vi "Main.vi"(11 "Module Admin":refnum<class "Delacor_lib_QMH_Module Admin.lvclass">) -> ()   [LabVIEW 2018, in "MB 01 switches Module.lvlib"]
doc: "This template is based off of the Queued Message Handler design pattern and the Queued Message Handler project template that ships with LabVIEW.\n\nThe main difference is that the queue is private to this module and communication between modules is performed via Broadcast and Request events.\n\nRequest events are wrapped in public API methods and are handled in the Event Handling Loop (EHL) of this VI. Any module can register for Broadcast events sent by this module. The EHL generates messages based on user interface actions.\n\nThe Message Handling Loop (MHL) processes messages generated by the EHL, or by other messages. The messages are string values, so new messages can be added easily to the Message Cases case structure in the MHL. Each message cluster can also provide an optional value for Message Data, which is a variant that can be converted to whatever message-specific data is required.\n_____\nBased on DQMH Project Template 6.0.0.91."
uses:
  MB 01 switches Module.lvlib
  <vilib>/Delacor/Delacor QMH/Libraries/Module Admin_class/Delacor_lib_QMH_Module Admin.lvclass
  Module Data--cluster.ctl
  <vilib>/NI/Modbus Library/API/Master/Modbus Master.lvclass
  <vilib>/Delacor/Delacor QMH/Libraries/Message Queue_class/Delacor_lib_QMH_Message Queue.lvclass/Delacor_lib_QMH_Message Queue.ctl
  Stop Argument--cluster.ctl
  <vilib>/Delacor/Delacor QMH/Libraries/Module Admin_class/Delacor_lib_QMH_Module Admin.lvclass/Delacor_lib_QMH_Module Admin.ctl
  MB01 Open Argument--cluster.ctl
  demux1-10 Argument--cluster.ctl
  MB01_eMICs Argument--cluster.ctl
  SC enable Argument--cluster.ctl
  MB01 Close Argument--cluster.ctl
  <vilib>/Utility/miscctls.llb/LVPointTypeDef.ctl
  <vilib>/Delacor/Delacor QMH/Libraries/Message Queue_class/Delacor_lib_QMH_Enqueue Message (Single).vi
  <vilib>/Delacor/Delacor QMH/Libraries/Module Admin_class/Delacor_lib_QMH_Get External Launch.vi
  <vilib>/Utility/error.llb/Error Cluster From Error Code.vi
  <vilib>/ErrorRing/Error Ring.xnode
  <vilib>/Delacor/Delacor QMH/Libraries/Message Queue_class/Delacor_lib_QMH_Message Queue.lvclass
  Instrument Drivers/LV_driver_MBrelay/MB Relay.lvlib
panel:
  out "error out":errorcluster
  out "Status":string
  in  "Simulate MHL Error":bool
  in  "Simulate EHL Error":bool
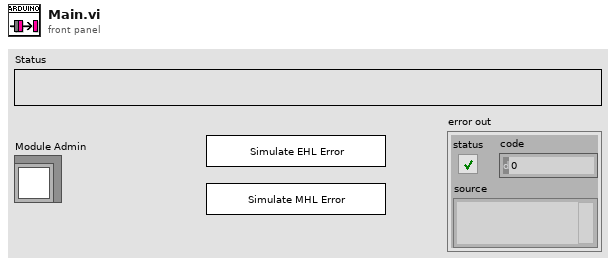
[diagram p1: front panel]
types:
  T1 = typedef "MB 01 switches Module.lvlib/Request Events--cluster.ctl" = cluster{"Stop Module":refnum<user-event>, "Show Panel":refnum<user-event>, "Hide Panel":refnum<user-event>, "Get Module Execution Status":refnum<user-event>, "Show Diagram":refnum<user-event>, "MB01 Open":refnum<user-event>, "demux1-10":refnum<user-event>, "MB01_eMICs":refnum<user-event>, "SC enable":refnum<user-event>, "MB01 Close":refnum<user-event>}
  T2 = typedef "MB 01 switches Module.lvlib/Module Data--cluster.ctl" = cluster{"Status":string, "VISA resource name":refnum<visa-resource-name>, "Modbus Master out":refnum<class "Modbus Master.lvclass">}
  T3 = enum32{"invalid lock state", "Not Locked", "Locked (No Password)", "Password-protected"}
  T4 = typedef "MB 01 switches Module.lvlib/Stop Argument--cluster.ctl" = cluster{"Origin":string, "Exit via Stop Module Req?":bool, "Wait for Module to stop?":bool}
  T5 = typedef "MB 01 switches Module.lvlib/MB01 Open Argument--cluster.ctl" = cluster{"VISA resource name":refnum<visa-resource-name>}
  T6 = typedef "MB 01 switches Module.lvlib/demux1-10 Argument--cluster.ctl" = cluster{"demux1_10(x6)_encode":enum16{"demux1_10_channel0", "demux1_10_channel1", "demux1_10_channel2", "demux1_10_channel3", "demux1_10_channel4", "demux1_10_channel5", "demux1_10_channel6", "demux1_10_channel7", "demux1_10_channel8", "demux1_10_channel9", "demux1_10_channel10"}}
  T7 = typedef "MB 01 switches Module.lvlib/MB01_eMICs Argument--cluster.ctl" = cluster{"Array":bool[]}
  T8 = typedef "MB 01 switches Module.lvlib/SC enable Argument--cluster.ctl" = cluster{"5V Enable":bool}
  T9 = typedef "MB 01 switches Module.lvlib/MB01 Close Argument--cluster.ctl" = cluster{"Boolean":bool}
  T10 = typedef "LVPointTypeDef.ctl" = cluster{"Horizontal":i16, "Vertical":i16}
  T11 = enum32{"Invalid", "Standard", "Closed", "Hidden", "Minimized", "Maximized"}
  T12 = enum16{"demux1_10_channel0", "demux1_10_channel1", "demux1_10_channel2", "demux1_10_channel3", "demux1_10_channel4", "demux1_10_channel5", "demux1_10_channel6", "demux1_10_channel7", "demux1_10_channel8", "demux1_10_channel9", "demux1_10_channel10"}
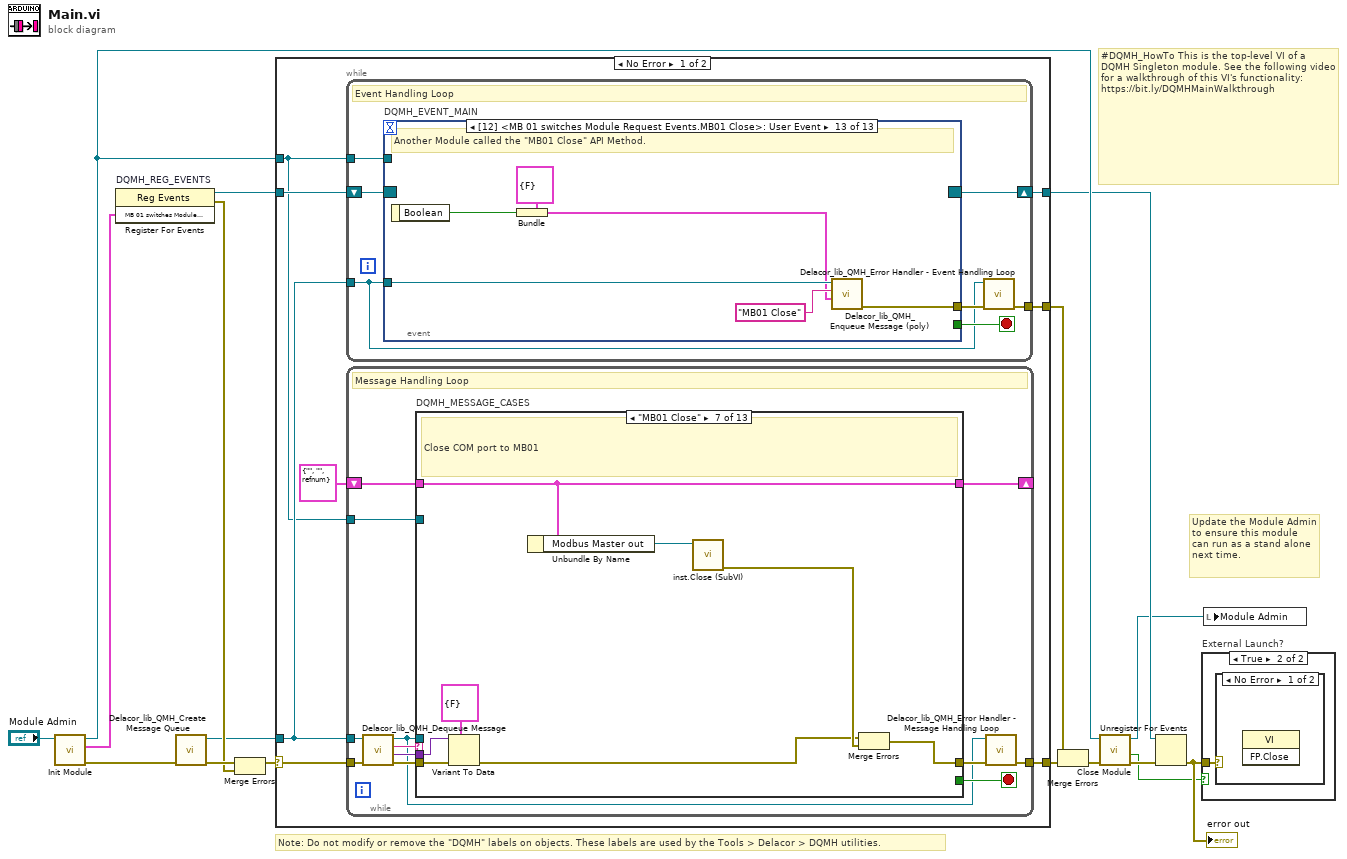
[diagram p0: block diagram]
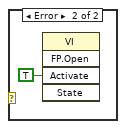
[diagram p3: hidden frame]
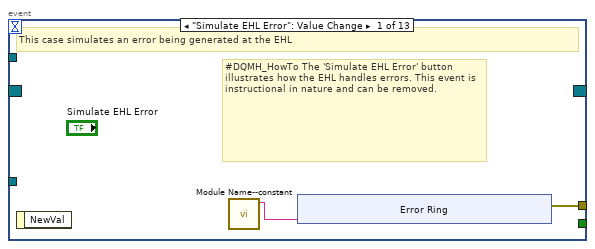
[diagram p4: hidden frame]
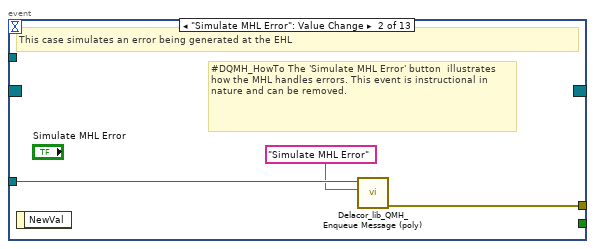
[diagram p5: hidden frame]
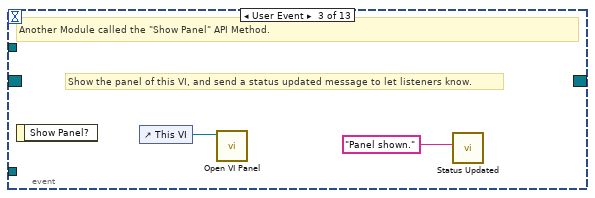
[diagram p6: hidden frame]
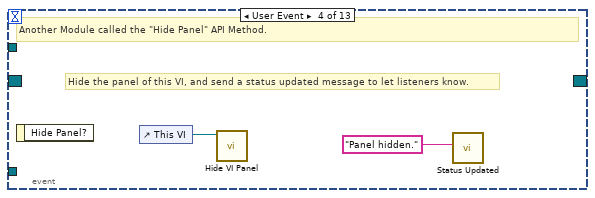
[diagram p7: hidden frame]
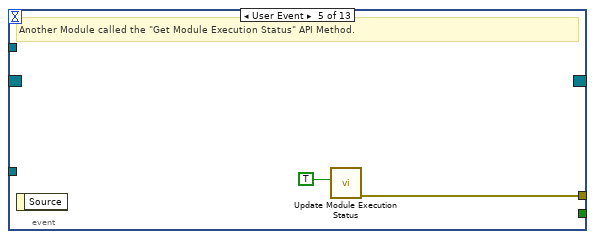
[diagram p8: hidden frame]
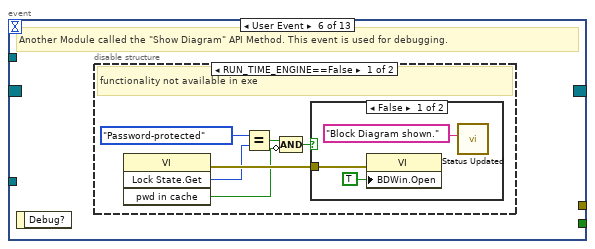
[diagram p9: hidden frame]
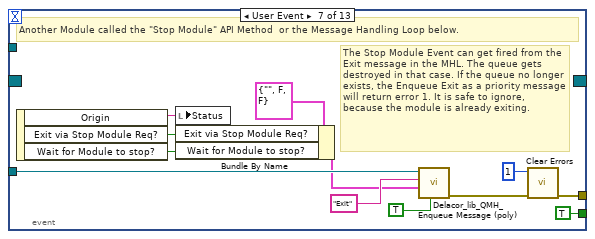
[diagram p12: hidden frame]
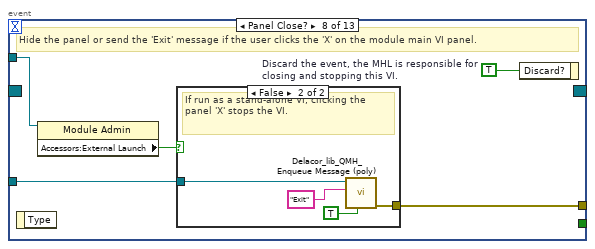
[diagram p13: hidden frame]
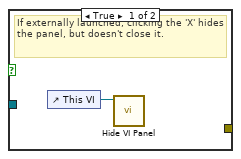
[diagram p14: hidden frame]
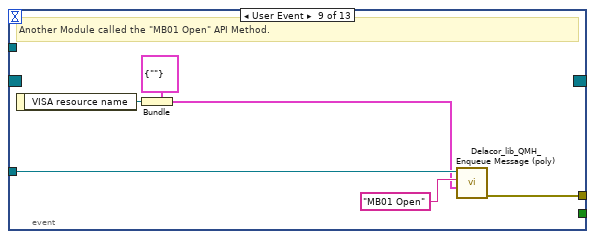
[diagram p15: hidden frame]
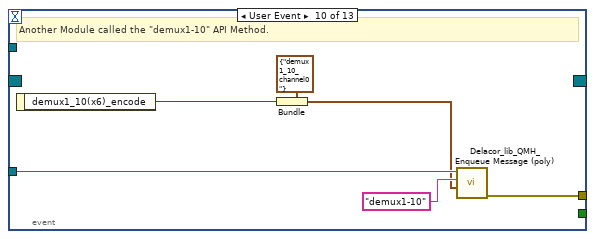
[diagram p16: hidden frame]
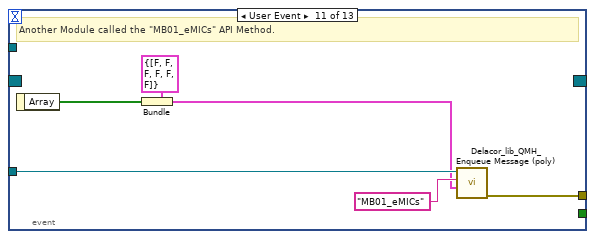
[diagram p17: hidden frame]
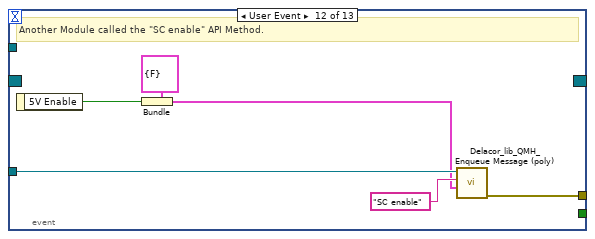
[diagram p18: hidden frame]
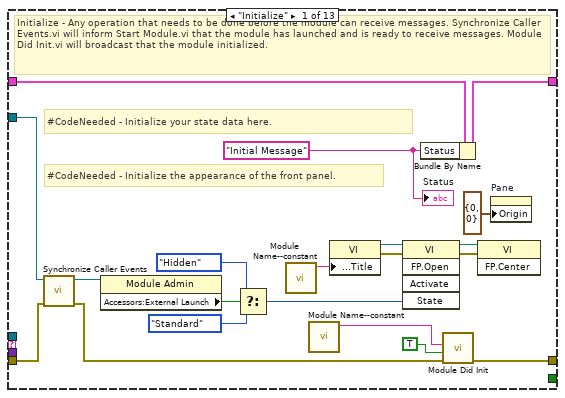
[diagram p19: hidden frame]
diagram:
  # "#DQMH_HowTo This is the top-level VI of a DQMH Singleton module. See the following video for a walkthrough of this VI's functionality: https://bit.ly/DQMHMainWalkthrough"
  # "Note: Do not modify or remove the \"DQMH\" labels on objects. These labels are used by the Tools > Delacor > DQMH utilities."
  # "Update the Module Admin to ensure this module can run as a stand alone next time."
  n1 = call "Init Module.vi"("Singleton Module Admin in"="Module Admin") -> ("error out"=w16:errorcluster, "MB 01 switches Module Request Events"=w5:T1, "Singleton Module Admin out"=w8:refnum<class "Delacor_lib_QMH_Module Admin.lvclass">)  [unwired: 8 in]
  n2 = register-events "DQMH_REG_EVENTS"(w5) -> (reference out=w6:refnum<event-registration>, error out=w9:errorcluster)  [unwired: 2 in]
  n3 = call <vilib>:"Delacor_lib_QMH_Create Message Queue.vi"("error in"=w16) -> ("error out"=w11:errorcluster, "Message Queue"=w4:refnum<class "Delacor_lib_QMH_Message Queue.lvclass">)  [unwired: 9 in]
  n4 = Merge Errors(w11, w9) -> (w10:errorcluster)
  n5 = case shown="No Error" w10 {
    selector: w10 -> [w23 w262]
    tunnel: [w25 w261] -> w17
    tunnel: [w22 w267] -> w7
    tunnel: w6 -> [w20 w267]
    tunnel: w4 -> [w19 w260]
    tunnel: [w24 _] -> w14
    tunnel: w8 -> [w18 w263]
    frame No Error {
      n6 = while {
        tunnel: w19 -> [w26]
        shift-right: [w29] -> w22
        shift-left: w20 -> [w30]
        tunnel: [w31] -> w24
        tunnel: w18 -> [w27]
        stop <- w28 stop-if-true
        # "Event Handling Loop"
        n7 = event "DQMH_EVENT_MAIN" shown="[12] <MB 01 switches Module Request Events.MB01 Close>: User Event" {
          selector: w30 -> [_ _ _ _ _ _ _ _ _ _ _ _ _]
          dyn-events: [_ _ _ _ _ _ _ _ _ _ _ _ _] -> w29
          timeout: _ -> [_ _ _ _ _ _ _ _ _ _ _ _ _]
          tunnel: [_ _ _ _ _ _ TRUE ("Discard?") _ _ _ _ _ _] -> w28
          tunnel: w26 -> [_ w43 _ _ _ _ w67 w74 w87 w93 w99 w105 w111]
          tunnel: [w34 w44 _ _ w50 _ w70 w76 w82 w88 w94 w100 w106] -> w32
          tunnel: w27 -> [_ _ _ _ _ _ _ w73 _ _ _ _ _]
          event "Simulate EHL Error": Value Change {
            # "#DQMH_HowTo The 'Simulate EHL Error' button  illustrates how the EHL handles errors. This event is instructional in nature and can be removed."
            # "This case simulates an error being generated at the EHL"
            n8 = event-data() -> ()  [unwired: 1 in, 1 out]
            n9 = call "Module Name--constant.vi"() -> ("Module Name"=w33:string)  [unwired: 11 in]
            n10 = xnode "Error Ring"("parameter 0"=w33) -> ("error out"=w34:errorcluster)
          }
          event "Simulate MHL Error": Value Change {
            # "#DQMH_HowTo The 'Simulate MHL Error' button  illustrates how the MHL handles errors. This event is instructional in nature and can be removed."
            # "This case simulates an error being generated at the EHL"
            n11 = event-data() -> ()  [unwired: 1 in, 1 out]
            n12 = call-poly <vilib>:"Delacor_lib_QMH_Enqueue Message (poly).vi"("Message"="Simulate MHL Error", "Message Queue in"=w43) -> ("error out"=w44:errorcluster)  [unwired: 8 in, 1 out]
          }
          event User Event {
            # "Show the panel of this VI, and send a status updated message to let listeners know."
            # "Another Module called the \"Show Panel\" API Method."
            n13 = event-data() -> ()  [unwired: 1 in, 1 out]
            n14 = control-ref of="This VI"() -> (w46:refnum<vi>)
            n15 = call "Open VI Panel.vi"("VI"=w46) -> ()  [unwired: 10 in, 1 out]
            n16 = call "Status Updated.vi"("Status"="Panel shown." ("format string")) -> ()  [unwired: 10 in, 1 out]
          }
          event User Event {
            # "Hide the panel of this VI, and send a status updated message to let listeners know."
            # "Another Module called the \"Hide Panel\" API Method."
            n17 = event-data() -> ()  [unwired: 1 in, 1 out]
            n18 = control-ref of="This VI"() -> (w48:refnum<vi>)
            n19 = call "Hide VI Panel.vi"("VI"=w48) -> ()  [unwired: 10 in, 1 out]
            n20 = call "Status Updated.vi"("Status"="Panel hidden." ("format string")) -> ()  [unwired: 10 in, 1 out]
          }
          event User Event {
            # "Another Module called the \"Get Module Execution Status\" API Method."
            n21 = event-data() -> ()  [unwired: 1 in, 1 out]
            n22 = call "Update Module Execution Status.vi"("Running?"=TRUE) -> ("error out"=w50:errorcluster)  [unwired: 10 in]
          }
          event User Event {
            # "Another Module called the \"Show Diagram\" API Method. This event is used for debugging."
            n23 = event-data() -> ()  [unwired: 1 in, 1 out]
            n24 = disable-structure shown="RUN_TIME_ENGINE==False" {
              frame condition #0 (active) {
                # "functionality not available in exe"
                n25 = invoke class="VI" method="Lock State.Get"() -> (error out=w56:errorcluster, "Get Lock State"=w55:T3, "pwd in cache"=w52:bool)  [unwired: 4 in, 1 out]
                n26 = Equal?(x=T3."Password-protected", y=w55) -> (x = y?=w53:bool)
                n27 = Compound Arithmetic op=AND(w53, invert w52) -> (w51:bool)
                n28 = case shown="False" w51 {
                  tunnel: w56 -> [w59 _]
                  frame False {
                    n29 = property class="VI"(error in=w59, "BDWin.Open"=TRUE ("Block Diagram Window:Open")) -> ()  [unwired: 1 in, 2 out]
                    n30 = call "Status Updated.vi"("Status"="Block Diagram shown." ("format string")) -> ()  [unwired: 10 in, 1 out]
                  }
                  frame True {
                    # "Password-protected VI, and the password is not in the cache. Do not show the diagram."
                  }
                }
              }
              frame condition #1 {
              }
            }
          }
          event User Event {
            # "The Stop Module Event can get fired from the Exit message in the MHL. The queue gets destroyed in that case. If the queue no longer exists, the Enqueue Exit as a priority message will return error 1. It is safe to ignore, because the module is already exiting."
            # "Another Module called the \"Stop Module\" API Method  or the Message Handling Loop below."
            n31 = event-data() -> ("Origin"=w66:string, "Exit via Stop Module Req?"=w62:bool, "Wait for Module to stop?"=w61:bool)  [unwired: 1 in]
            n32 = local write "Status"(w66) -> ()
            n33 = Bundle By Name(cluster=T4 {"Origin"="", "Exit via Stop Module Req?"=FALSE, "Wait for Module to stop?"=FALSE} ("Stop Argument"), "Exit via Stop Module Req?"=w62, "Wait for Module to stop?"=w61) -> (w60:T4)
            n34 = call-poly <vilib>:"Delacor_lib_QMH_Enqueue Message (poly).vi"("Priority Message? (F)"=TRUE, "Message Data"=w60, "Message"="Exit", "Message Queue in"=w67) -> ("error out"=w71:errorcluster)  [unwired: 6 in, 1 out]
            n35 = call <vilib>:"Clear Errors.vi"("error in (no error)"=w71, "specific error code to clear (0: all)"=1) -> ("error out"=w70:errorcluster)  [unwired: 4 in, 1 out]
          }
          event Panel Close? {
            w75 = TRUE  # Discard the event, the MHL is responsible for closing and stopping this VI.
            # "Hide the panel or send the 'Exit' message if the user clicks the 'X' on the module main VI panel."
            n36 = event-data() -> ()  [unwired: 1 in, 1 out]
            n37 = property class="Module Admin"(reference=w73) -> ("Accessors:External Launch"=w72:bool)  [unwired: 1 in, 2 out]
            n38 = case shown="False" w72 {
              tunnel: w74 -> [_ w80]
              tunnel: [_ w81] -> w76
              frame True {
                # "If externally launched, clicking the 'X' hides the panel, but doesn't close it."
                n39 = control-ref of="This VI"() -> (w77:refnum<vi>)
                n40 = call "Hide VI Panel.vi"("VI"=w77) -> ()  [unwired: 10 in, 1 out]
              }
              frame False {
                # "If run as a stand-alone VI, clicking the panel 'X' stops the VI."
                n41 = call-poly <vilib>:"Delacor_lib_QMH_Enqueue Message (poly).vi"("Priority Message? (F)"=TRUE, "Message"="Exit", "Message Queue in"=w80) -> ("error out"=w81:errorcluster)  [unwired: 7 in, 1 out]
              }
            }
            n42 = event-data("Discard?"=w75) -> ()  [unwired: 1 in, 1 out]
          }
          event User Event {
            # "Another Module called the \"MB01 Open\" API Method."
            n43 = event-data() -> ("VISA resource name"=w83:refnum<visa-resource-name>)  [unwired: 1 in]
            n44 = Bundle(cluster=T5 {"VISA resource name"=""} ("MB01 Open Argument"), "VISA resource name"=w83) -> (w84:T5)
            n45 = call-poly <vilib>:"Delacor_lib_QMH_Enqueue Message (poly).vi"("Message Data"=w84, "Message"="MB01 Open", "Message Queue in"=w87) -> ("error out"=w82:errorcluster)  [unwired: 7 in, 1 out]
          }
          event User Event {
            # "Another Module called the \"demux1-10\" API Method."
            n46 = event-data() -> ("demux1_10(x6)_encode"=w89:T12)  [unwired: 1 in]
            n47 = Bundle(cluster=T6 {"demux1_10(x6)_encode"=enum."demux1_10_channel0"} ("demux1-10 Argument"), "demux1_10(x6)_encode"=w89) -> (w90:T6)
            n48 = call-poly <vilib>:"Delacor_lib_QMH_Enqueue Message (poly).vi"("Message Data"=w90, "Message"="demux1-10", "Message Queue in"=w93) -> ("error out"=w88:errorcluster)  [unwired: 7 in, 1 out]
          }
          event User Event {
            # "Another Module called the \"MB01_eMICs\" API Method."
            n49 = event-data() -> ("Array"=w95:bool[])  [unwired: 1 in]
            n50 = Bundle(cluster=T7 {"Array"=[FALSE, FALSE, FALSE, FALSE, FALSE, FALSE]} ("MB01_eMICs Argument"), "Array"=w95) -> (w96:T7)
            n51 = call-poly <vilib>:"Delacor_lib_QMH_Enqueue Message (poly).vi"("Message Data"=w96, "Message"="MB01_eMICs", "Message Queue in"=w99) -> ("error out"=w94:errorcluster)  [unwired: 7 in, 1 out]
          }
          event User Event {
            # "Another Module called the \"SC enable\" API Method."
            n52 = event-data() -> ("5V Enable"=w101:bool)  [unwired: 1 in]
            n53 = Bundle(cluster=T8 {"5V Enable"=FALSE} ("SC enable Argument"), "5V Enable"=w101) -> (w102:T8)
            n54 = call-poly <vilib>:"Delacor_lib_QMH_Enqueue Message (poly).vi"("Message Data"=w102, "Message"="SC enable", "Message Queue in"=w105) -> ("error out"=w100:errorcluster)  [unwired: 7 in, 1 out]
          }
          event User Event {
            # "Another Module called the \"MB01 Close\" API Method."
            n55 = event-data() -> ("Boolean"=w107:bool)  [unwired: 1 in]
            n56 = Bundle(cluster=T9 {"Boolean"=FALSE} ("MB01 Close Argument"), "Boolean"=w107) -> (w108:T9)
            n57 = call-poly <vilib>:"Delacor_lib_QMH_Enqueue Message (poly).vi"("Message Data"=w108, "Message"="MB01 Close", "Message Queue in"=w111) -> ("error out"=w106:errorcluster)  [unwired: 7 in, 1 out]
          }
        }
        n58 = call-dynamic "Delacor_lib_QMH_Error Handler - Event Handling Loop.vi"("error in"=w32, "Message Queue in"=w26) -> ("dup error in"=w31:errorcluster)  [unwired: 8 in, 1 out]
      }
      n59 = while {
        tunnel: w19 -> [w114]
        shift-right: [w118] -> _
        shift-left: T2 {"Status"="", "VISA resource name"="", "Modbus Master out"=refnum} ("Data Cluster") -> [w119]
        tunnel: w23 -> [w122]
        tunnel: [w120] -> w25
        tunnel: w18 -> [w112]
        stop <- w117 stop-if-true
        # "Message Handling Loop"
        n60 = call-dynamic "Delacor_lib_QMH_Dequeue Message.vi"("error in"=w122, "Message Queue in"=w114) -> ("error out"=w121:errorcluster, "Message Data"=w115:variant, "Message"=w116:string, "Message Queue out"=w113:refnum<class "Delacor_lib_QMH_Message Queue.lvclass">)  [unwired: 6 in]
        n61 = case "DQMH_MESSAGE_CASES" shown="\"MB01 Close\"" w116 {
          selector: w116 -> [_ _ _ _ _ _ _ _ _ _ _ _ w247]
          tunnel: w113 -> [_ _ _ _ _ _ _ _ _ _ w215 w239 _]
          tunnel: w121 -> [w141 w145 w157 w167 w177 w187 w195 w198 w200 w205 w222 w245 w249]
          tunnel: [w139 w145 w146 w158 w168 w180 w188 w197 w200 w204 w218 w242 w250] -> w123
          tunnel: w119 -> [w130 w144 w149 w163 w173 w183 w192 w196 w199 w202 w217 w231 w248]
          tunnel: [w129 w144 w150 w163 w173 w183 w192 w196 w199 w202 w217 w231 w248] -> w118
          tunnel: [_ _ _ _ _ _ _ _ _ _ _ w238 _] -> w117
          tunnel: w115 -> [_ _ w156 w166 w176 w186 w194 _ _ _ w216 w237 _]
          tunnel: w112 -> [w131 _ _ _ _ _ _ _ _ _ w214 w232 _]
          frame "Initialize" {
            w125 = "Initial Message" ("Initial Message")
            # "#CodeNeeded - Initialize the appearance of the front panel."
            # "#CodeNeeded - Initialize your state data here."
            # "Initialize - Any operation that needs to be done before the module can receive messages. Synchronize Caller Events.vi will inform Start Module.vi that the module has launched and is ready to receive messages. Module Did Init.vi will broadcast that the module initialized."
            n62 = call "Synchronize Caller Events.vi"("error in (no error)"=w141, "Singleton Module Admin in"=w131) -> ("error out"=w140:errorcluster, "Singleton Module Admin out"=w126:refnum<class "Delacor_lib_QMH_Module Admin.lvclass">)  [unwired: 8 in]
            n63 = property class="Module Admin"(reference=w126) -> ("Accessors:External Launch"=w135:bool)  [unwired: 1 in, 2 out]
            n64 = Select(t=T11."Hidden" ("State"), s=w135, f=T11."Standard" ("State")) -> (s? t:f=w132:T11)
            n65 = call "Module Name--constant.vi"() -> ("Module Name"=w138:string)  [unwired: 11 in]
            n66 = call "Module Name--constant.vi"() -> ("Module Name"=w127:string)  [unwired: 11 in]
            n67 = property class="VI"("Front Panel.Title"=w138) -> (reference out=w137:refnum<vi>, error out=w143:errorcluster)  [unwired: 2 in]
            n68 = invoke class="VI" method="FP.Open"(reference=w137, error in=w143, "State"=w132) -> (reference out=w136:refnum<vi>, error out=w142:errorcluster)  [unwired: 2 in, 3 out]
            n69 = Bundle By Name(cluster=w130, "Status"=w125) -> (w129:T2)
            n70 = call "Module Did Init.vi"("error in (no error)"=w140, "Initialized?"=TRUE, "Origin"=w127) -> ("error out"=w139:errorcluster)  [unwired: 8 in]
            n71 = invoke class="VI" method="FP.Center"(reference=w136, error in=w142) -> ()  [unwired: 1 in, 3 out]
            n72 = property on="Pane" class="Pane"("Origin"=T10 {"Horizontal"=0, "Vertical"=0}) -> ()  [unwired: 2 in, 2 out]
            "Status" <- w125
          }
          frame "---Module Specific---" {
            # "Separator -- The following cases handle messages specific to this Module."
          }
          frame "MB01 Open" {
            # "Open mobus on MB01"
            n73 = Variant To Data(error in=w157, type=T5 {"VISA resource name"=""} ("MB01 Open Argument"), Variant=w156) -> (data=w154:T5, error out=w147:errorcluster)
            n74 = Unbundle By Name(w154) -> ("VISA resource name"=w153:refnum<visa-resource-name>)
            n75 = call "inst.Open.vi"("unit ID in"=u8 1, "VISA resource name"=w153) -> ("error out"=w148:errorcluster, "Modbus Master out"=w151:refnum<class "Modbus Master.lvclass">)  [unwired: 8 in]
            n76 = Bundle By Name(cluster=w149, "Modbus Master out"=w151) -> (w150:T2)
            n77 = Merge Errors(w147, w148) -> (w146:errorcluster)
          }
          frame "demux1-10" {
            # "Control demux 1-10 ( AC switches)"
            n78 = Variant To Data(error in=w167, type=T6 {"demux1_10(x6)_encode"=enum."demux1_10_channel0"} ("demux1-10 Argument"), Variant=w166) -> (data=w164:T6, error out=w159:errorcluster)
            n79 = Unbundle By Name(w163) -> ("Modbus Master out"=w162:refnum<class "Modbus Master.lvclass">)
            n80 = Unbundle By Name(w164) -> ("demux1_10(x6)_encode"=w161:T12)
            n81 = call "inst.demux1.10(x6).vi"("demux1_10(x6)_encode"=w161, "Modbus Master in"=w162) -> ("error out"=w160:errorcluster)  [unwired: 8 in, 1 out]
            n82 = Merge Errors(w159, w160) -> (w158:errorcluster)
          }
          frame "MB01_eMICs" {
            # "MB01 TurnON/OFF eMICs ( connect AC220V)"
            n83 = Variant To Data(error in=w177, type=T7 {"Array"=[FALSE, FALSE, FALSE, FALSE, FALSE, FALSE]} ("MB01_eMICs Argument"), Variant=w176) -> (data=w174:T7, error out=w169:errorcluster)
            n84 = Unbundle By Name(w174) -> ("Array"=w171:bool[])
            n85 = Unbundle By Name(w173) -> ("Modbus Master out"=w172:refnum<class "Modbus Master.lvclass">)
            n86 = call "inst.MB Relay01(eMICs).vi"("MB relay01"=w171, "Modbus Master in"=w172) -> ("error out"=w170:errorcluster)  [unwired: 8 in, 1 out]
            n87 = Merge Errors(w169, w170) -> (w168:errorcluster)
          }
          frame "SC enable" {
            # "Enable 5V to check Shorted Circuit of Led DRV"
            n88 = Variant To Data(error in=w187, type=T8 {"5V Enable"=FALSE} ("SC enable Argument"), Variant=w186) -> (data=w184:T8, error out=w181:errorcluster)
            n89 = Unbundle By Name(w183) -> ("Modbus Master out"=w182:refnum<class "Modbus Master.lvclass">)
            n90 = Unbundle By Name(w184) -> ("5V Enable"=w178:bool)
            n91 = call "inst.SC enable.vi"("5V enable"=w178, "Modbus Master in"=w182) -> ("error out"=w179:errorcluster)  [unwired: 8 in, 1 out]
            n92 = Merge Errors(w181, w179) -> (w180:errorcluster)
          }
          frame "MB01 Close" {
            # "Close COM port to MB01"
            n93 = Variant To Data(error in=w195, type=T9 {"Boolean"=FALSE} ("MB01 Close Argument"), Variant=w194) -> (error out=w189:errorcluster)  [unwired: 1 out]
            n94 = Unbundle By Name(w192) -> ("Modbus Master out"=w191:refnum<class "Modbus Master.lvclass">)
            n95 = call "inst.Close (SubVI).vi"("Modbus Master in"=w191) -> ("error out"=w190:errorcluster)  [unwired: 10 in]
            n96 = Merge Errors(w189, w190) -> (w188:errorcluster)
          }
          frame "---Copy This Frame---" {
            # "Duplicate this frame when creating new messages.  Change this comment in the duplicated frame to describe this message."
            n97 = Merge Errors(w198) -> (w197:errorcluster)
          }
          frame "---Exit and Error Handling---" {
            # "Separator - The following cases handle errors and exit messages."
          }
          frame "Simulate MHL Error" {
            # "#DQMH_HowTo The 'Simulate MHL Error' button  illustrates how the MHL handles errors. This event is instructional in nature and can be removed."
            # "Simulate an error occurring at the MHL"
            n98 = call "Module Name--constant.vi"() -> ("Module Name"=w201:string)  [unwired: 11 in]
            n99 = xnode "Error Ring"("parameter 0"=w201) -> ("error out"=w203:errorcluster)
            n100 = Merge Errors(w205, w203) -> (w204:errorcluster)
          }
          frame "Error" {
            # "#CodeRecommended - If you ever change the name of this \"Error\" message, you'll need to update the name in the Check Loop Error.vi as well."
            # "#CodeRecommended - If the module is running in standalone mode (External Launch = FALSE), this code will pop up an error dialog and call the 'Exit' message if an error occurs. Add more fine-grained error handling here."
            # "Error - Check the error message data and respond accordingly. This message is sent by the \"Error Handler\" VIs at the end of each loop in this application."
            n101 = property class="Module Admin"(reference=w214) -> ("Accessors:External Launch"=w213:bool)  [unwired: 1 in, 2 out]
            n102 = Variant To Data(error in=w222, type=errorcluster {"status"=FALSE, "code"=0, "source"=""} ("error constant"), Variant=w216) -> (data=w223:errorcluster, error out=w220:errorcluster)
            n103 = call "Error Reported.vi"("Error"=w223) -> ()  [unwired: 10 in, 1 out]
            n104 = case shown="False" w213 {
              tunnel: [w228 _] -> w219
              tunnel: w215 -> [w226 _]
              tunnel: w223 -> [w227 _]
              frame False {
                # "If the module is running standalone, then pop up an error dialog and call the \"Exit\" message."
                n105 = call <vilib>:"Simple Error Handler.vi"("error in (no error)"=w227) -> ()  [unwired: 4 in, 5 out]
                n106 = call-poly <vilib>:"Delacor_lib_QMH_Enqueue Message (poly).vi"("Priority Message? (F)"=TRUE, "Message"="Exit", "Message Queue in"=w226) -> ("error out"=w228:errorcluster)  [unwired: 7 in, 1 out]
              }
              frame True {
                # "If the module was launched externally, calling the Error Reported broadcast VI is the only action performed by the \"Error\" message. The module's caller can then process the error appropriately."
              }
            }
            n107 = Merge Errors(w220, w219) -> (w218:errorcluster)
            n108 = local write "error out"(w218) -> ()
          }
          frame "Exit" {
            w236 = 91  # 91: not all Exit messages will have an argument
            w238 = TRUE  # Stop the VI
            # "Release the message queue reference"
            # "Exit - Exit the application."
            n109 = Variant To Data(error in=w245, type=T4 {"Origin"="", "Exit via Stop Module Req?"=FALSE, "Wait for Module to stop?"=FALSE} ("Stop Argument"), Variant=w237) -> (data=w234:T4, error out=w241:errorcluster)
            n110 = Unbundle By Name(w231) -> ("Modbus Master out"=w230:refnum<class "Modbus Master.lvclass">)
            n111 = call <vilib>:"Clear Errors.vi"("error in (no error)"=w241, "specific error code to clear (0: all)"=w236) -> ("error out"=w244:errorcluster)  [unwired: 4 in, 1 out]
            n112 = control-ref of="This VI"() -> (w233:refnum<vi>)
            n113 = call "Handle Exit.vi"("Stop Argument"=w234, "Admin in"=w232, "VI reference"=w233) -> ("error out"=w240:errorcluster)  [unwired: 7 in, 1 out]
            n114 = call "inst.Close (SubVI).vi"("Modbus Master in"=w230) -> ("error out"=w229:errorcluster)  [unwired: 10 in]
            n115 = call-dynamic "Delacor_lib_QMH_Release Message Queue.vi"("error in"=w244, "Message Queue"=w239) -> ("error out"=w243:errorcluster)  [unwired: 9 in]
            n116 = Merge Errors(w243, w240, w229) -> (w242:errorcluster)
          }
          frame Default {
            # "'Default' case only runs if there is a message that isn't defined in any of the other cases.  Output a programming error."
            n117 = call "Module Name--constant.vi"() -> ("Module Name"=w246:string)  [unwired: 11 in]
            n118 = xnode "Error Ring"("parameter 0"=w247, "parameter 1"=w246) -> ("error out"=w251:errorcluster)
            n119 = Merge Errors(w249, w251) -> (w250:errorcluster)
          }
        }
        n120 = call-dynamic "Delacor_lib_QMH_Error Handler - Message Handling Loop.vi"("error in"=w123, "Message Queue in"=w113) -> ("dup error in"=w120:errorcluster)  [unwired: 8 in, 1 out]
      }
    }
    frame Error {
      # "Synchronize Caller Events.vi will inform Start Module.vi that the module has launched and will let the code calling Start Module.vi register for broadcasts and would permit the caller receive the broadcast that an error occurred at launch time."
      n121 = call-dynamic "Delacor_lib_QMH_Release Message Queue.vi"("error in"=w262, "Message Queue"=w260) -> ("error out"=w261:errorcluster)  [unwired: 9 in]
      n122 = call "Synchronize Caller Events.vi"("Singleton Module Admin in"=w263) -> ("error out"=w268:errorcluster)  [unwired: 9 in, 1 out]
      n123 = call "Module Name--constant.vi"() -> ("Module Name"=w266:string)  [unwired: 11 in]
      n124 = Format Into String(format string="An error occurred during initialization. %s is no longer running.", w266) -> (resulting string=w264:string)  [unwired: 2 in, 1 out]
      n125 = Merge Errors(w261, w268) -> (w269:errorcluster)
      n126 = call "Error Reported.vi"("Additional Information"=w264, "Error"=w269) -> ()  [unwired: 9 in, 1 out]
    }
  }
  n127 = Merge Errors(w14, w17) -> (w13:errorcluster)
  n128 = call "Close Module.vi"("error in (no error)"=w13, "Module Admin in"=w8) -> ("error out"=w15:errorcluster, "External Launch"=w1:bool, "Module Admin out"=w2:refnum<class "Delacor_lib_QMH_Module Admin.lvclass">)  [unwired: 7 in]
  n129 = Unregister For Events(event registration refnum=w7, error in=w15) -> (error out=w12:errorcluster)
  "error out" <- w12
  n130 = case "External Launch?" shown="True" w1 {
    tunnel: w12 -> [_ w270]
    frame False {
    }
    frame True {
      n131 = case shown="No Error" w270 {
        frame No Error {
          n132 = invoke class="VI" method="FP.Close"() -> ()  [unwired: 3 in, 3 out]
        }
        frame Error {
          n133 = invoke class="VI" method="FP.Open"("Activate"=TRUE ("Activate?")) -> ()  [unwired: 4 in, 5 out]
        }
      }
    }
  }
  n134 = local write "Module Admin"(w2) -> ()
